vi "5.1.-Detección de Bordes Sobel y Prewitt.vi"() -> ()   [LabVIEW 2020]
panel:
  in  "stop":bool
  in  "Enum":enum16{"PREWITT", "SOBEL"}(ring)
  out "Detección de Bordes":enum32{"SOBEL", "PREWITT"}(tab)
  out "Sobel Gx":picture
  out "Sobel Gy":picture
  out "Sobel G":picture
  out "Prewitt Gy":picture
  out "Prewitt Gx":picture
  out "Prewitt G":picture
  in  "Path":path
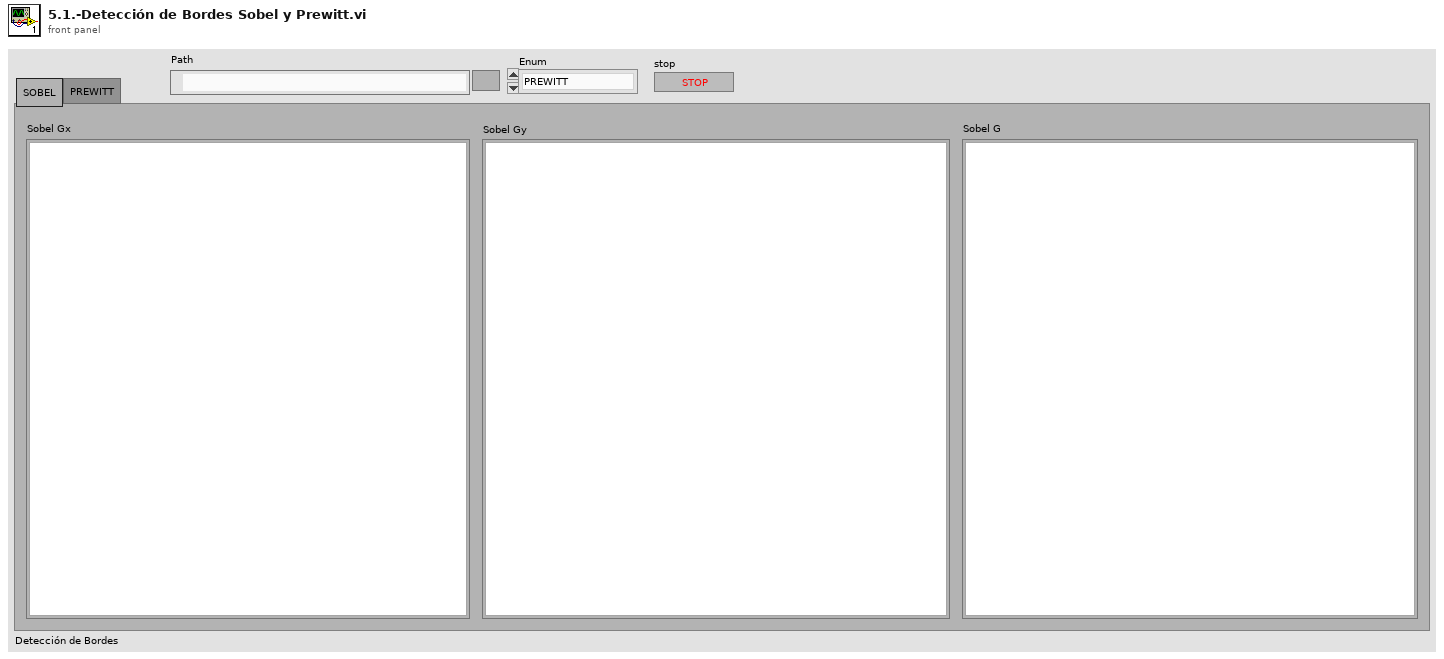
[diagram p1: front panel]
types:
  T1 = typedef "imagedata.ctl" = cluster{"image type":i32, "image depth":i32, "image":u8[], "mask":u8[], "colors":u32[], "Rectangle":cluster{"left":i16, "top":i16, "right":i16, "bottom":i16}}
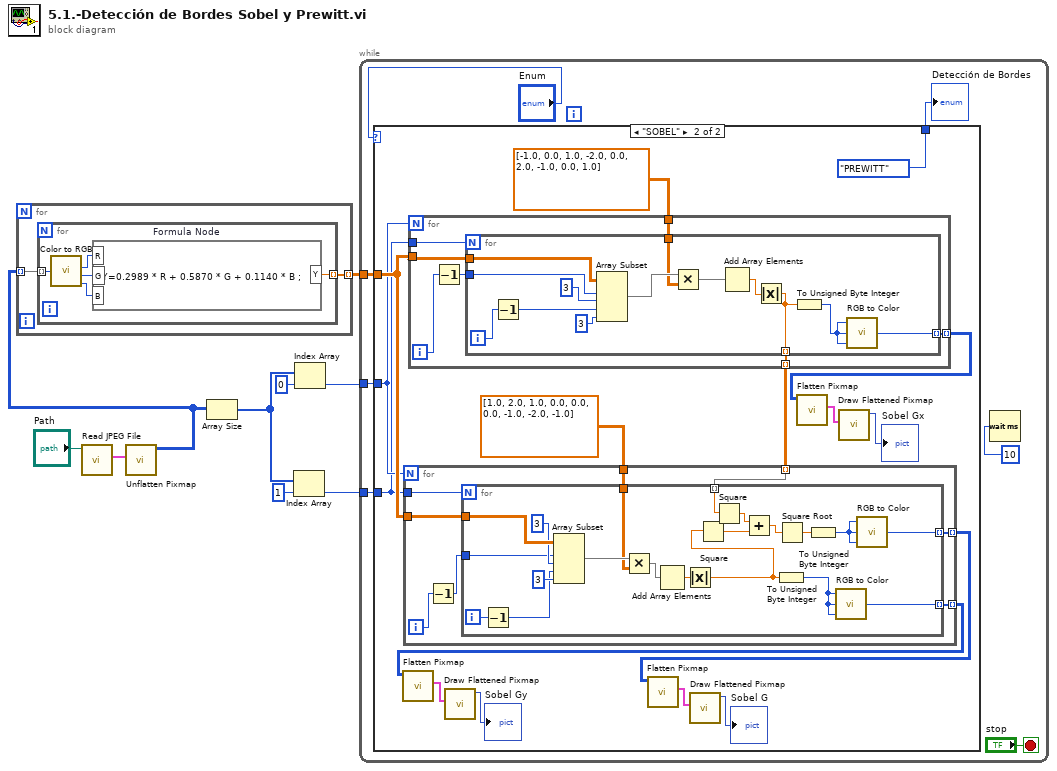
[diagram p0: block diagram]
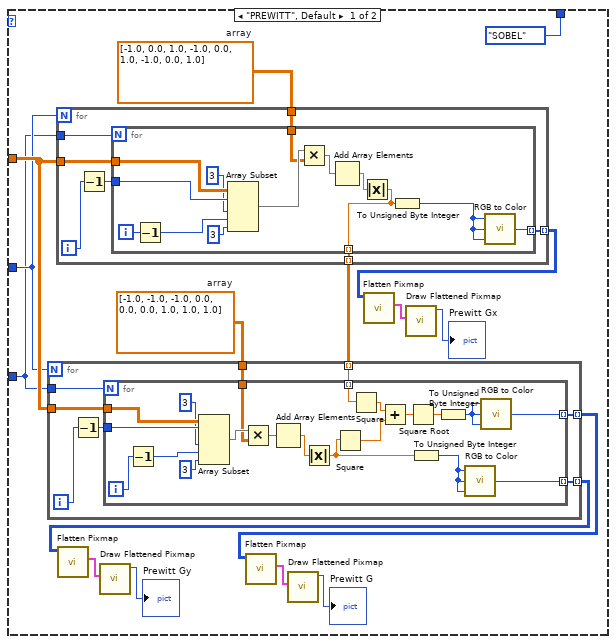
[diagram p2: hidden frame]
diagram:
  n1 = call <vilib>:"Read JPEG File.vi"("path to JPEG file"="Path") -> ("image data"=w8:T1)  [unwired: 8 in, 2 out]
  n2 = call <vilib>:"Unflatten Pixmap.vi"("image data"=w8) -> ("24-bit pixmap"=w6:u32[][])  [unwired: 4 in, 6 out]
  n3 = for {
    tunnel: w6 -> [w11] mode=indexing
    tunnel: [w10] -> w7 mode=indexing
    n4 = for {
      tunnel: w11 -> [w16] mode=indexing
      tunnel: [w12] -> w10 mode=indexing
      n5 = call <vilib>:"Color to RGB.vi"("Color"=w16) -> ("R"=w15:u8, "G"=w14:u8, "B"=w13:u8)  [unwired: 1 out]
      n6 = formula code="Y=0.2989 * R + 0.5870 * G + 0.1140 * B ;"("R"=w15, "G"=w14, "B"=w13) -> ("Y"=w12:dbl)
    }
  }
  n7 = Array Size(array=w6) -> (size(s)=w4:i32[])
  n8 = Index Array "Index Array"(array=w4, index=1) -> (element=w1:i32)
  n9 = Index Array "Index Array"(array=w4, index=0) -> (element=w2:i32)
  n10 = while {
    tunnel: w7 -> [w23]
    tunnel: w2 -> [w19]
    tunnel: w1 -> [w18]
    stop <- "stop" stop-if-true
    n11 = case shown="\"SOBEL\"" "Enum" {
      tunnel: w23 -> [w33 w97]
      tunnel: w19 -> [w28 w92]
      tunnel: w18 -> [w27 w91]
      tunnel: [enum32{"SOBEL", "PREWITT"}."SOBEL" ("Tab Control") enum32{"SOBEL", "PREWITT"}."PREWITT" ("Tab Control")] -> w17
      frame "PREWITT", Default {
        w25 = dbl[][] [[-1.0, -1.0, -1.0], [0.0, 0.0, 0.0], [1.0, 1.0, 1.0]]  # array
        w26 = dbl[][] [[-1.0, 0.0, 1.0], [-1.0, 0.0, 1.0], [-1.0, 0.0, 1.0]]  # array
        n12 = for {
          N: w28 -> [_]
          tunnel: w33 -> [w74]
          tunnel: w26 -> [w71]
          tunnel: [w70] -> w38 mode=indexing
          tunnel: [w69] -> w32 mode=indexing
          tunnel: w27 -> [w68]
          i -> [w73]
          n13 = Decrement(x=w73) -> (x-1=w72:i32)
          n14 = for {
            N: w68 -> [_]
            tunnel: w74 -> [w87]
            tunnel: w72 -> [w77]
            tunnel: w71 -> [w83]
            tunnel: [w79] -> w70 mode=indexing
            tunnel: [w78] -> w69 mode=indexing
            i -> [w85]
            n15 = Decrement(x=w85) -> (x-1=w86:i32)
            n16 = Array Subset "Array Subset"(array=w87, index (row)=w77, length (row)=3 ("length"), index (col)=w86, length (col)=3 ("length")) -> (w84:dbl[][])
            n17 = Multiply(x=w84, y=w83) -> (x*y=w82:dbl[][])
            n18 = Add Array Elements(numeric array=w82) -> (sum=w81:dbl)
            n19 = Absolute Value(x=w81) -> (abs(x)=w78:dbl)
            n20 = To Unsigned Byte Integer(number=w78) -> (unsigned 8bit integer=w80:u8)
            n21 = call <vilib>:"RGB to Color.vi"("B"=w80, "G"=w80, "R"=w80) -> ("Color"=w79:u32)
          }
        }
        n22 = for {
          N: w28 -> [_]
          tunnel: w33 -> [w47]
          tunnel: w25 -> [w44]
          tunnel: [w43] -> w36 mode=indexing
          tunnel: [w42] -> w30 mode=indexing
          tunnel: w32 -> [w41] mode=indexing
          tunnel: w27 -> [w40]
          i -> [w46]
          n23 = Decrement(x=w46) -> (x-1=w45:i32)
          n24 = for {
            N: w40 -> [_]
            tunnel: w47 -> [w67]
            tunnel: w45 -> [w57]
            tunnel: w44 -> [w65]
            tunnel: [w61] -> w43 mode=indexing
            tunnel: [w59] -> w42 mode=indexing
            tunnel: w41 -> [w51] mode=indexing
            i -> [w55]
            n25 = Decrement(x=w55) -> (x-1=w56:i32)
            n26 = Array Subset "Array Subset"(array=w67, index (row)=w57, length (row)=3 ("length"), index (col)=w56, length (col)=3 ("length")) -> (w66:dbl[][])
            n27 = Multiply(x=w66, y=w65) -> (x*y=w64:dbl[][])
            n28 = Add Array Elements(numeric array=w64) -> (sum=w63:dbl)
            n29 = Absolute Value(x=w63) -> (abs(x)=w49:dbl)
            n30 = Square(x=w49) -> (x^2=w48:dbl)
            n31 = Square(x=w51) -> (x^2=w50:dbl)
            n32 = Add(x=w50, y=w48) -> (x+y=w58:dbl)
            n33 = Square Root(x=w58) -> (sqrt(x)=w60:dbl)
            n34 = To Unsigned Byte Integer(number=w49) -> (unsigned 8bit integer=w62:u8)
            n35 = To Unsigned Byte Integer(number=w60) -> (unsigned 8bit integer=w52:u8)
            n36 = call <vilib>:"RGB to Color.vi"("B"=w62, "G"=w62, "R"=w62) -> ("Color"=w61:u32)
            n37 = call <vilib>:"RGB to Color.vi"("B"=w52, "G"=w52, "R"=w52) -> ("Color"=w59:u32)
          }
        }
        n38 = call <vilib>:"Flatten Pixmap.vi"("24-bit pixmap"=w36) -> ("image data"=w37:T1)  [unwired: 10 in]
        n39 = call <vilib>:"Draw Flattened Pixmap.vi"("image data"=w37) -> ("new picture"=→"Prewitt Gy":picture)  [unwired: 8 in]
        n40 = call <vilib>:"Flatten Pixmap.vi"("24-bit pixmap"=w30) -> ("image data"=w31:T1)  [unwired: 10 in]
        n41 = call <vilib>:"Draw Flattened Pixmap.vi"("image data"=w31) -> ("new picture"=→"Prewitt G":picture)  [unwired: 8 in]
        n42 = call <vilib>:"Flatten Pixmap.vi"("24-bit pixmap"=w38) -> ("image data"=w39:T1)  [unwired: 10 in]
        n43 = call <vilib>:"Draw Flattened Pixmap.vi"("image data"=w39) -> ("new picture"=→"Prewitt Gx":picture)  [unwired: 8 in]
      }
      frame "SOBEL" {
        n44 = for {
          N: w92 -> [_]
          tunnel: w97 -> [w138]
          tunnel: dbl[][] [[-1.0, 0.0, 1.0], [-2.0, 0.0, 2.0], [-1.0, 0.0, 1.0]] ("array") -> [w137]
          tunnel: [w136] -> w101 mode=indexing
          tunnel: [w135] -> w94 mode=indexing
          tunnel: w91 -> [w134]
          i -> [w133]
          n45 = Decrement(x=w133) -> (x-1=w132:i32)
          n46 = for {
            N: w134 -> [_]
            tunnel: w138 -> [w151]
            tunnel: w137 -> [w148]
            tunnel: [w144] -> w136 mode=indexing
            tunnel: [w143] -> w135 mode=indexing
            tunnel: w132 -> [w139]
            i -> [w150]
            n47 = Decrement(x=w150) -> (x-1=w140:i32)
            n48 = Array Subset "Array Subset"(array=w151, index (row)=w139, length (row)=3 ("length"), index (col)=w140, length (col)=3 ("length")) -> (w149:dbl[][])
            n49 = Multiply(x=w149, y=w148) -> (x*y=w147:dbl[][])
            n50 = Add Array Elements(numeric array=w147) -> (sum=w146:dbl)
            n51 = Absolute Value(x=w146) -> (abs(x)=w143:dbl)
            n52 = To Unsigned Byte Integer(number=w143) -> (unsigned 8bit integer=w145:u8)
            n53 = call <vilib>:"RGB to Color.vi"("B"=w145, "G"=w145, "R"=w145) -> ("Color"=w144:u32)
          }
        }
        n54 = for {
          N: w92 -> [_]
          tunnel: w97 -> [w111]
          tunnel: dbl[][] [[1.0, 2.0, 1.0], [0.0, 0.0, 0.0], [-1.0, -2.0, -1.0]] ("array") -> [w110]
          tunnel: [w109] -> w98 mode=indexing
          tunnel: [w108] -> w95 mode=indexing
          tunnel: w94 -> [w107] mode=indexing
          tunnel: w91 -> [w106]
          i -> [w105]
          n55 = Decrement(x=w105) -> (x-1=w104:i32)
          n56 = for {
            N: w106 -> [_]
            tunnel: w111 -> [w131]
            tunnel: w110 -> [w129]
            tunnel: [w125] -> w109 mode=indexing
            tunnel: [w122] -> w108 mode=indexing
            tunnel: w107 -> [w115] mode=indexing
            tunnel: w104 -> [w117]
            i -> [w121]
            n57 = Decrement(x=w121) -> (x-1=w118:i32)
            n58 = Array Subset "Array Subset"(array=w131, index (row)=w117, length (row)=3 ("length"), index (col)=w118, length (col)=3 ("length")) -> (w130:dbl[][])
            n59 = Multiply(x=w130, y=w129) -> (x*y=w128:dbl[][])
            n60 = Add Array Elements(numeric array=w128) -> (sum=w127:dbl)
            n61 = Absolute Value(x=w127) -> (abs(x)=w112:dbl)
            n62 = Square(x=w112) -> (x^2=w113:dbl)
            n63 = Square(x=w115) -> (x^2=w114:dbl)
            n64 = Add(x=w114, y=w113) -> (x+y=w123:dbl)
            n65 = To Unsigned Byte Integer(number=w112) -> (unsigned 8bit integer=w126:u8)
            n66 = Square Root(x=w123) -> (sqrt(x)=w124:dbl)
            n67 = To Unsigned Byte Integer(number=w124) -> (unsigned 8bit integer=w116:u8)
            n68 = call <vilib>:"RGB to Color.vi"("B"=w126, "G"=w126, "R"=w126) -> ("Color"=w125:u32)
            n69 = call <vilib>:"RGB to Color.vi"("B"=w116, "G"=w116, "R"=w116) -> ("Color"=w122:u32)
          }
        }
        n70 = call <vilib>:"Flatten Pixmap.vi"("24-bit pixmap"=w98) -> ("image data"=w100:T1)  [unwired: 10 in]
        n71 = call <vilib>:"Draw Flattened Pixmap.vi"("image data"=w100) -> ("new picture"=→"Sobel Gy":picture)  [unwired: 8 in]
        n72 = call <vilib>:"Flatten Pixmap.vi"("24-bit pixmap"=w95) -> ("image data"=w96:T1)  [unwired: 10 in]
        n73 = call <vilib>:"Draw Flattened Pixmap.vi"("image data"=w96) -> ("new picture"=→"Sobel G":picture)  [unwired: 8 in]
        n74 = call <vilib>:"Flatten Pixmap.vi"("24-bit pixmap"=w101) -> ("image data"=w103:T1)  [unwired: 10 in]
        n75 = call <vilib>:"Draw Flattened Pixmap.vi"("image data"=w103) -> ("new picture"=→"Sobel Gx":picture)  [unwired: 8 in]
      }
    }
    "Detección de Bordes" <- w17
    n76 = Wait (ms)(milliseconds to wait=u32 10) -> ()  [unwired: 1 out]
  }
